vi "Add Header.vi"(8 "error in (no error)":errorcluster, 11 "Text File Sink in":refnum<class "Text File Sink.lvclass">) -> (0 "error out":errorcluster, 3 "Text File Sink out":refnum<class "Text File Sink.lvclass">)   [LabVIEW 2016, in "Stream Log.lvlib" / "Text File Sink.lvclass"]
doc: "--\nCopyright © 2017 Composed SystemsI All rights reserved.\n\nAuthor: Jon McBee <jon.mcbee@composed.io>\n\nThis library is provided \"AS IS\" ,WITHOUT WARRANTIES OR\nCONDITIONS OF ANY KIND, either express or implied.\n\nComposed Systems -- composed.io\n\nStream 0.0.1.1\nJon McBee - Composed Systems\nCopyright (c) 2017, Composed Systems"
uses:
  <userlib>/Composed Systems/Stream/Log/Text File Sink/Text File Sink.lvclass
  <userlib>/Composed Systems/Stream/Log/Text File Sink/Text File Sink.lvclass/Text File Sink.ctl
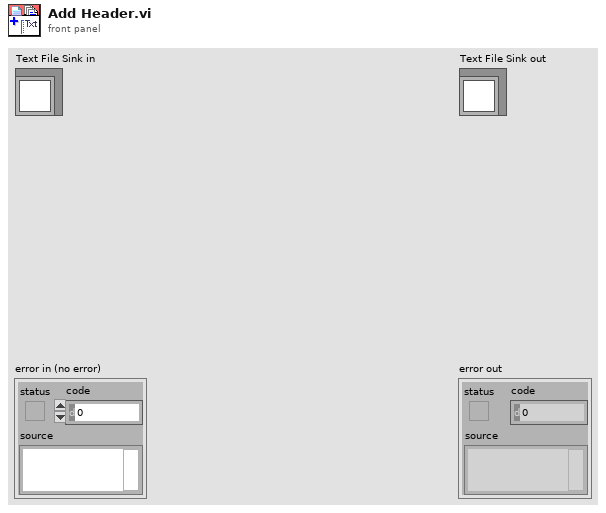
[diagram p1: front panel]
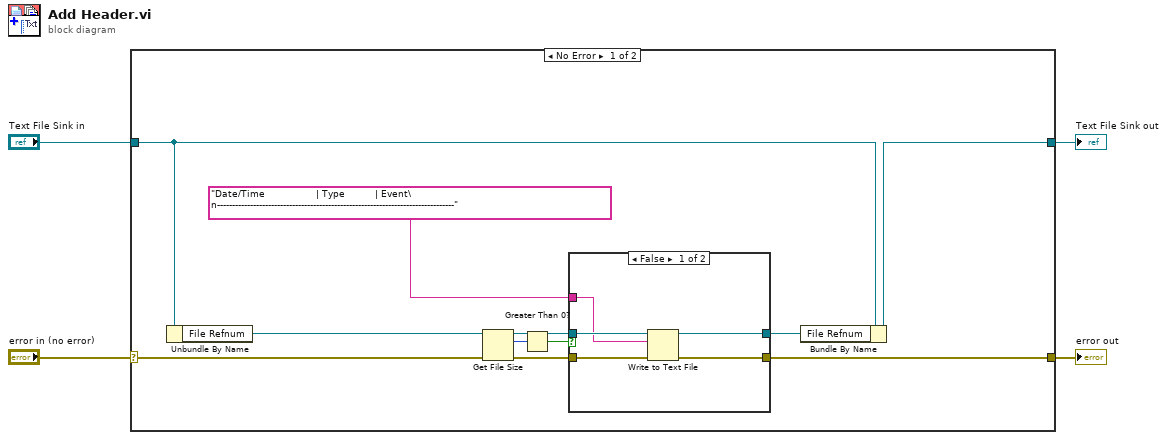
[diagram p0: block diagram]
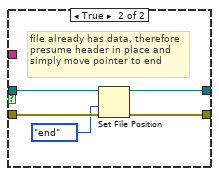
[diagram p2: hidden frame]
diagram:
  n1 = case shown="No Error" "error in (no error)" {
    selector: "error in (no error)" -> [w9 w27]
    tunnel: [w7 w27] -> w3
    tunnel: [w8 w26] -> w1
    tunnel: "Text File Sink in" -> [w6 w26]
    frame No Error {
      n2 = Unbundle By Name(w6) -> ("File Refnum"=w11:refnum<file>)
      n3 = Get File Size(file=w11, error in=w9) -> (refnum out=w12:refnum<file>, size (in bytes)=w15:i64, 0:w14:errorcluster)
      n4 = Greater Than 0?(x=w15) -> (x > 0?=w13:bool)
      n5 = case shown="False" w13 {
        tunnel: w14 -> [w20 w25]
        tunnel: w12 -> [w19 w24]
        tunnel: [w16 w22] -> w7
        tunnel: [w17 w21] -> w10
        tunnel: "Date/Time                 | Type          | Event\n-------------------------------------------------------------------------------" ("File Header") -> [w18 _]
        frame False {
          n6 = Write to Text File(file (use dialog)=w19, text=w18, error in=w20) -> (refnum out=w17:refnum<file>, error out=w16:errorcluster)  [unwired: 2 out]
        }
        frame True {
          # "file already has data, therefore\npresume header in place and\nsimply move pointer to end"
          n7 = Set File Position(refnum=w24, from (0:start)=enum16{"start", "end", "current"}."end", error in=w25) -> (refnum out=w21:refnum<file>, error out=w22:errorcluster)  [unwired: 1 out]
        }
      }
      n8 = Bundle By Name(cluster=w6, "File Refnum"=w10) -> (w8:refnum<class "Text File Sink.lvclass">)
    }
    frame Error {
    }
  }
  "error out" <- w3
  "Text File Sink out" <- w1
